vi "HovaCal Komm.vi"() -> (0 "error IO":errorcluster)   [LabVIEW 2020, in "Linearisierung v2.lvlib" / "Gasteiler.lvlib" / "HovaCal.lvlib"]
uses:
  HovaCal.lvlib
  Aktion_FGV_Kom.ctl
  Aktionen FGV Gasteiler Daten.ctl
  Daten abholen.ctl
  Aktion unterbrechen.ctl
  HovaCAL_Interface/Kommunikation/Aktion_FGV_HovaCAL_Interface_Kommunikation.ctl
  HovaCAL_Interface/Kommunikation/Aktion_FGV_HovaCAL_Interface_Kommandos.ctl
  Aktion FGV Stoerungen sammeln und auswerten.ctl
  Gasteiler.lvlib
  Linearisierung v2.lvlib
  Aktion FGV Rohmesswerte sammeln.ctl
  Aktion_FGV_Betriebsdaten.ctl
  Aktion Lin Daten aufarbeiten.ctl
  HovaCAL_Interface/Kommunikation/Kommunikation.lvlib
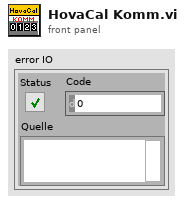
[diagram p1: front panel]
types:
  T1 = typedef "Linearisierung v2.lvlib/Gasteiler.lvlib/Aktion unterbrechen.ctl" = enum16{"Betrieb", "Unterbrechen", "Warten"}
  T2 = typedef "Linearisierung v2.lvlib/Daten abholen.ctl" = enum16{"Initialisieren", "Punkt aufschalten", "Warten", "Daten abholen", "Fertig", "Beenden", "Spülen", "Abbrechen"}
  T3 = typedef "Linearisierung v2.lvlib/Gasteiler.lvlib/Aktionen FGV Gasteiler Daten.ctl" = enum16{"lesen", "Gasteiler Daten", "Seriellen Param.", "MB-Endwert", "laden", "speichern", "Anforderung", "TCP", "Aufzeichnung Start"}
  T4 = typedef "Linearisierung v2.lvlib/Gasteiler.lvlib/HovaCal.lvlib/Aktion_FGV_Kom.ctl" = enum16{"Initialisieren", "Betriebsparameter", "Gase", "Vaporizer", "Dynamische Werte", "Beenden", "Com ändern", "Gase init"}
  T5 = typedef "Linearisierung v2.lvlib/Gasteiler.lvlib/HovaCAL_Interface.lvlib/Kommunikation.lvlib/Aktion_FGV_HovaCAL_Interface_Kommunikation.ctl" = enum16{"Initialisieren", "Set Konzentrationen", "Set Gase", "Set Limits", "Get Dynamische Werte", "Beenden", "Com ändern", "Get Gase init", "Pause", "Get Gasteiler Infos", "Get MFC Infos", "Set Pumpen Parameter", "Set Pumpe Konzenration", "Set Pumpe run", "Set Temperaturen", "Set Fluss", "Get Gase", "Get Limits", "Get Dynamische Werte 1", "Get Dynamische Werte 2"}
  T6 = typedef "Linearisierung v2.lvlib/Gasteiler.lvlib/HovaCAL_Interface.lvlib/Kommunikation.lvlib/Aktion_FGV_HovaCAL_Interface_Kommandos.ctl" = enum16{"lesen", "verarbeiten", "hinzufügen", "on top", "init", "sammeln", "freigeben", "connected"}
  T7 = typedef "Linearisierung v2.lvlib/Aktion Lin Daten aufarbeiten.ctl" = enum16{"lesen", "Protkolldaten", "speichern", "laden", "EPA auswerten", "Tabelle schreiben", "Lin auswerten", "Tab init", "Stufentabelle", "EPA aktiviert", "Nachbehandlung laden", "Tabelle löschen", "Istwerte löschen", "Zeile löschen", "Zeile einfügen", "LIN aktiviert", "LIN/EPA aktiv laden", "EGAK Tab", "LIN übernehmen", "Tab init ohne Stufen"}
  T8 = typedef "Linearisierung v2.lvlib/Gasteiler.lvlib/HovaCal.lvlib/Aktion_FGV_Betriebsdaten.ctl" = enum16{"Lesen", "Sollwerte schreiben", "Sollwerte lesen", "Gase schreiben", "Gase lesen", "Dynamische Werte", "GaseRef", "Gase aendern"}
  T9 = typedef "Linearisierung v2.lvlib/Aktion FGV Rohmesswerte sammeln.ctl" = enum16{"lesen", "schreiben", "löschen", "Sollwert HovaCal"}
  T10 = typedef "Linearisierung v2.lvlib/Aktion FGV Stoerungen sammeln und auswerten.ctl" = enum16{"init", "lesen", "error", "prüfen", "reset error", "abbrechen", "fortsetzen", "neustart", "Bedientasten reset"}
  T11 = typedef "Linearisierung v2.lvlib/Gasteiler.lvlib/Gasteiler Daten.ctl" = cluster{"Gasteiler":T12, "Gasteiler Stufen":T13, "Gasteiler Type":T14, "Konfig Gasteiler":T15, "Gasteiler Span Eingänge":u16}
  T12 = typedef "String - Eingabefeld.ctl" = string
  T13 = typedef "Linearisierung v2.lvlib/Gasteiler.lvlib/Gasteiler Stufen.ctl" = u16
  T14 = typedef "Linearisierung v2.lvlib/GasteilerType.ctl" = u16
  T15 = typedef "System Einstellungen V2.lvlib/Gasteiler Auswahl.ctl" = u16
  T16 = typedef "Linearisierung v2.lvlib/Lin-Polynom Daten.ctl" = cluster{"Messgerät":string, "Kalibrator (Gasteiler)":string, "Bearbeiter/in":string, "Komponente":string, "Zeitstempel":timestamp, "F_max gefordert (%)":sgl, "F_max in %":sgl, "F_max in ppm":sgl, "Vorschlag Ordnung":i32, "Polynom OK":bool, "Polynomkoeff.":dbl[], "Prüfgas Konzentration":dbl, "Pfad EPA":string, "Pfad_LIN":string, "Gasnummer:":u8, "Komponentenauswahl":T17, "Verdünnungsgas":T19, "Zeitdauer Stufe":T20, "Anzahl Stufen":T20, "F_max in % EPA":sgl, "F_max in ppm EPA":sgl, "F_max in % LIN":sgl, "F_max in ppm LIN":sgl, "Punkte umkehren":bool, "EPA Optionsfeld":T21, "Autolin Hovacal":T22, "Spanfactors":sgl[], "Kalibrierauswahl":T23, "Conditions:":T24, "Gasflaschen Nr.:":string, "Bottle Accuracy":dbl, "Konfig Gasflasche":T25, "Gasflasche":T26, "HovaCAL Flow AutoLin":T27, "MFC Output":T28, "Gas Ablaufdatum":timestamp, "Lin Modus":T29, "zusätzliche Zeitdauer Erster Punkt":sgl, "Offsets":sgl[]}
  T17 = typedef "Linearisierung v2.lvlib/KomponentenArray.ctl" = cluster{"Komponente:":T18, "Konzentration":dbl}[]
  T18 = typedef "Auswahlfeld.ctl" = u16
  T19 = typedef "Linearisierung v2.lvlib/Gasteiler.lvlib/Prüfgas in.ctl" = u16
  T20 = typedef "Zahlen-Eingabefeld.ctl" = sgl
  T21 = typedef "Linearisierung v2.lvlib/EPA Optionsfeld.ctl" = enum32{"Istwert", "Rohwert", "Linearisierter Wert"}
  T22 = typedef "Linearisierung v2.lvlib/Gasteiler.lvlib/HovaCal.lvlib/AutoLin Hovacal.ctl" = enum32{"Keine Auswahl", "Optionsauswahl 1", "Optionsauswahl 2"}
  T23 = typedef "Linearisierung v2.lvlib/Kalibrieroption.ctl" = u16
  T24 = typedef "Linearisierung v2.lvlib/Linearity verification 1065-307.lvlib/Condition.ctl" = u16
  T25 = typedef "System Einstellungen V2.lvlib/Konfig Gasflasche.ctl" = bool
  T26 = typedef "System Einstellungen V2.lvlib/Gasflasche Auswahl.ctl" = u16
  T27 = typedef "Linearisierung v2.lvlib/Gasteiler.lvlib/HovaCAL_Interface.lvlib/Controls.lvlib/Flow Einstellung.ctl" = cluster{"HovaCAL Flow Input Cluster":dbl}
  T28 = typedef "Linearisierung v2.lvlib/Gasteiler.lvlib/HovaCAL_Interface.lvlib/Controls.lvlib/Pump state.ctl" = cluster{"Run":bool}
  T29 = typedef "CalGas Aufschaltung.lvlib/Lin Modus.ctl" = u16
  T30 = typedef "Linearisierung v2.lvlib/Gasteiler.lvlib/HovaCal.lvlib/Dynamsiche_Werte.ctl" = cluster{"Durchfluss":dbl, "Drehzahl":dbl, "Wasserkonz.":dbl, "Ist - Temp":dbl, "Ist Konz 1":dbl, "Ist Konz 2":dbl}
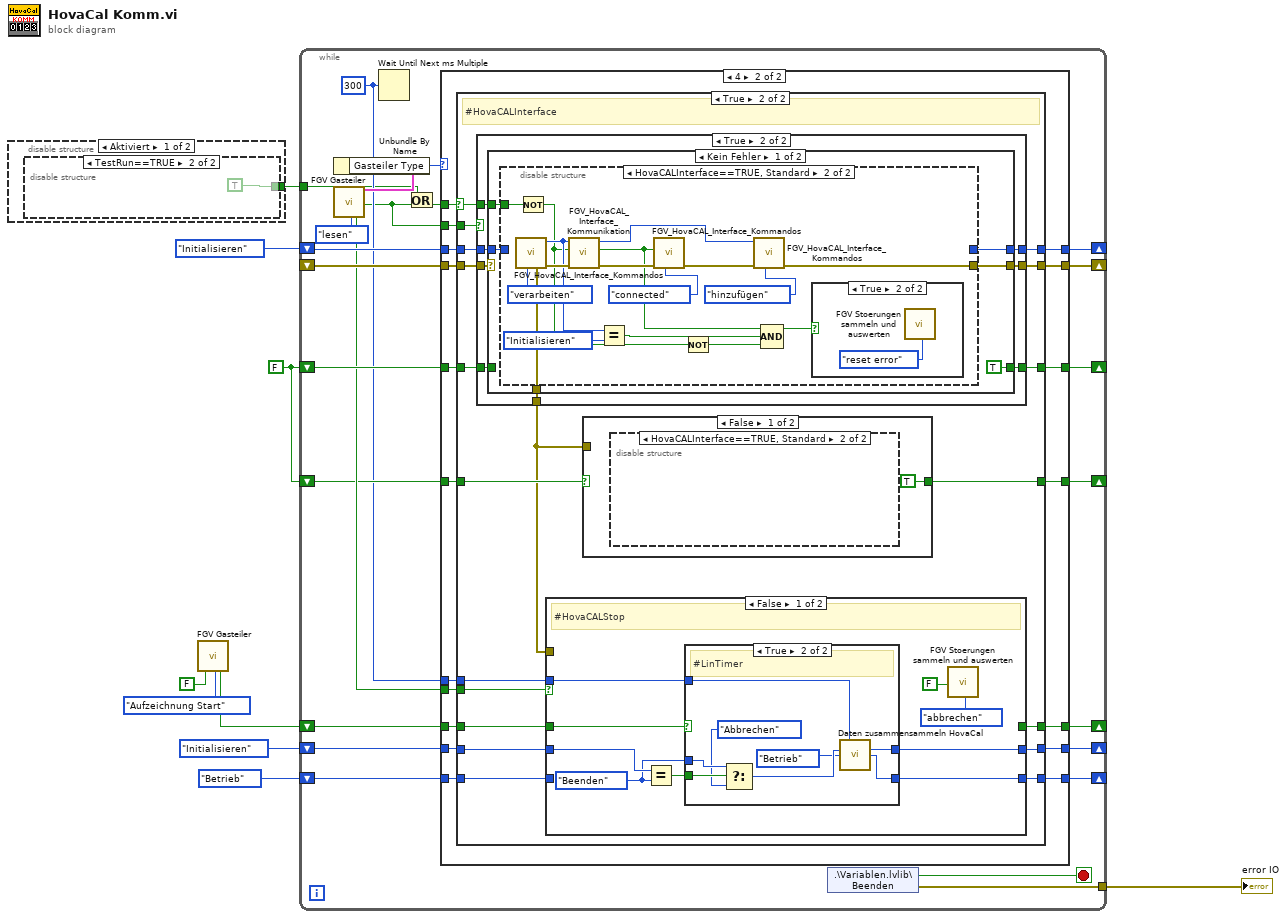
[diagram p0: block diagram]
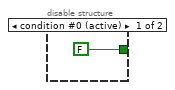
[diagram p2: hidden frame]
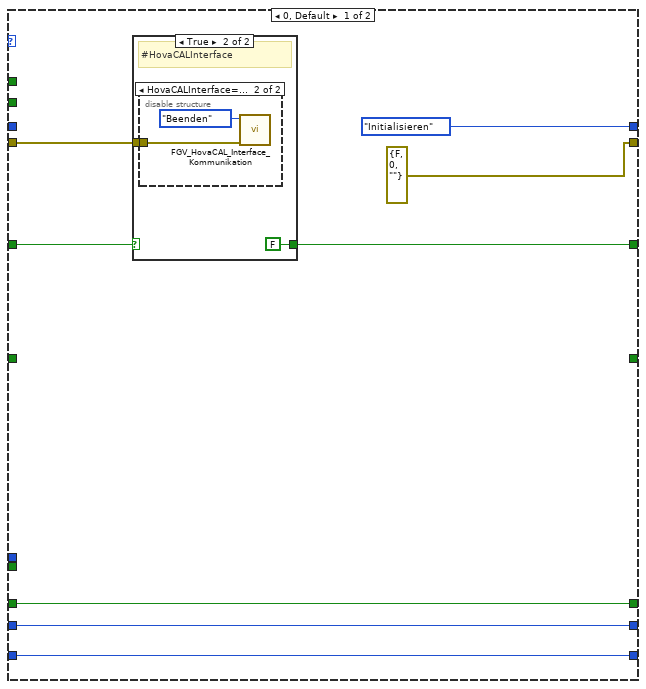
[diagram p4: hidden frame]
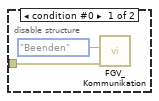
[diagram p6: hidden frame]
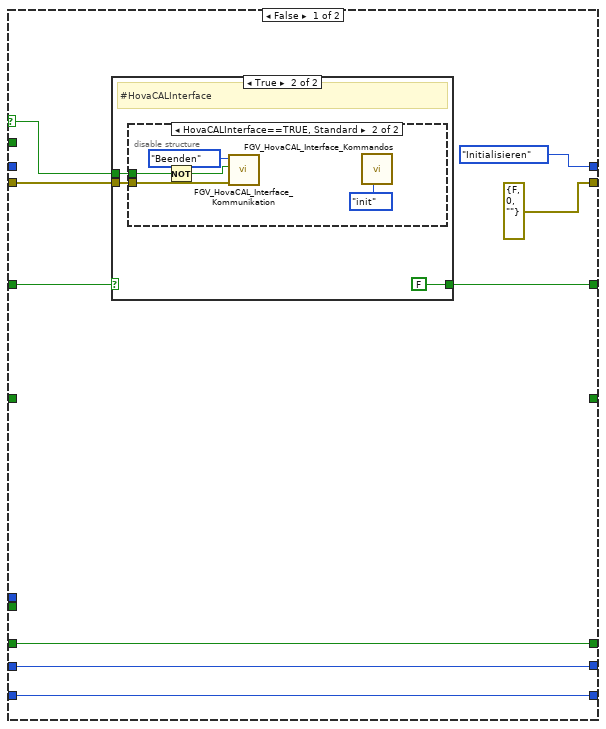
[diagram p7: hidden frame]
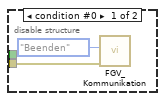
[diagram p9: hidden frame]
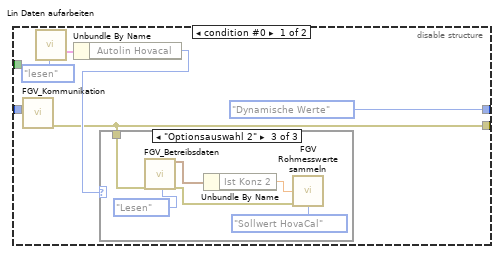
[diagram p11: hidden frame]
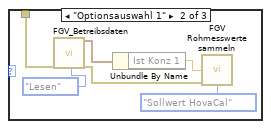
[diagram p13: hidden frame]
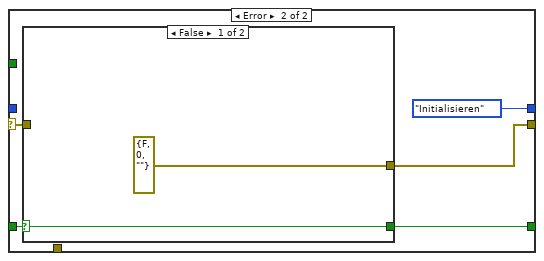
[diagram p15: hidden frame]
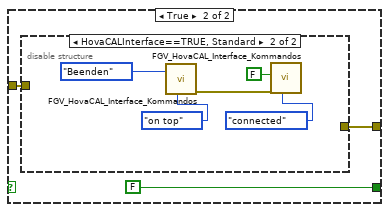
[diagram p16: hidden frame]
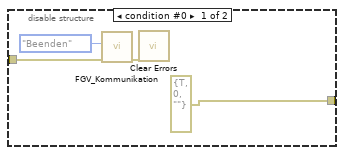
[diagram p17: hidden frame]
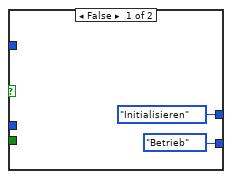
[diagram p18: hidden frame]
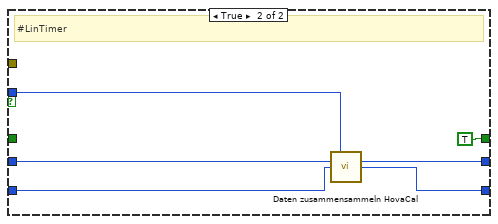
[diagram p19: hidden frame]
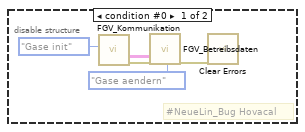
[diagram p20: hidden frame]
diagram:
  w4 = FALSE
  n1 = disable-structure shown="Aktiviert" {
    disable-tunnel: [w10 _] -> w2
    frame Enabled {
      n2 = disable-structure shown="TestRun==TRUE" {
        disable-tunnel: [FALSE TRUE] -> w10
        frame condition #0 (active) {
        }
        frame condition #1 {
        }
      }
    }
    frame Disabled {
    }
  }
  n3 = call "FGV Gasteiler.vi"("Aufzeichnung Start"=FALSE, "Aktionen"=Aktionen_FGV_Gasteiler_Daten."Aufzeichnung Start") -> ("Aufzeichnung Start"=w5:bool)  [unwired: 10 in, 7 out]
  n4 = while {
    shift-right: [w35] -> _
    shift-left: Aktion_FGV_Kom."Initialisieren" ("Aktion") -> [w36]
    shift-right: [w33] -> _
    shift-left: _ -> [w32]
    tunnel: [w30] -> w8
    shift-right: [w27] -> _
    shift-left: w4 -> [w28]
    shift-right: [w26] -> _
    shift-left: w5 -> [w25]
    shift-right: [w23] -> _
    shift-left: Daten_abholen."Initialisieren" ("Aktionen Daten abholen") -> [w24]
    shift-right: [w20] -> _
    shift-left: w4 -> [w21]
    tunnel: w2 -> [w16]
    shift-right: [w13] -> _
    shift-left: Aktion_unterbrechen."Betrieb" ("Aktion Unterbrechen") -> [w14]
    stop <- w31 stop-if-true
    w18 = u32 300 ("Vielfache von ms")
    n5 = call "FGV Gasteiler.vi"("Aktionen"=Aktionen_FGV_Gasteiler_Daten."lesen") -> ("Aufzeichnung Start"=w22:bool, "Gasteiler Daten"=w29:T11, "Anforderung"=w15:bool)  [unwired: 11 in, 5 out]
    n6 = Unbundle By Name(w29) -> ("Gasteiler Type"=w19:T14)
    n7 = Wait Until Next ms Multiple(millisecond multiple=w18) -> ()  [unwired: 1 out]
    n8 = Or(x=w16, y=w15) -> (x .or. y?=w17:bool)
    n9 = case shown="4" w19 {
      tunnel: w36 -> [_ w69]
      tunnel: [Aktion_FGV_Kom."Initialisieren" ("Aktion") w68] -> w35
      tunnel: w17 -> [_ w67]
      tunnel: [errorcluster {"status"=FALSE, "code"=0, "source"=""} ("error out") w66] -> w33
      tunnel: w32 -> [w40 w65]
      tunnel: w28 -> [w42 w64]
      tunnel: [w41 w63] -> w27
      tunnel: [w39 w56] -> w26
      tunnel: w25 -> [w39 w58]
      tunnel: w24 -> [w38 w59]
      tunnel: [w38 w57] -> w23
      tunnel: w22 -> [_ w60]
      tunnel: w21 -> [_ w62]
      tunnel: [_ w61] -> w20
      tunnel: w18 -> [_ w55]
      tunnel: w15 -> [_ w54]
      tunnel: w14 -> [w37 w53]
      tunnel: [w37 w52] -> w13
      frame 0, Default {
        n10 = case shown="True" w42 {
          selector: w42 -> [w45 _]
          tunnel: w40 -> [_ w47]
          tunnel: [w45 FALSE] -> w41
          frame False {
          }
          frame True {
            # "#HovaCALInterface"
            n11 = disable-structure shown="HovaCALInterface==TRUE, Standard" {
              disable-tunnel: w47 -> [w49 w50]
              frame condition #0 {
                n12 = call "FGV_Kommunikation.vi"("error in"=w49, "Aktion"=Aktion_FGV_Kom."Beenden") -> ()  [unwired: 5 in, 5 out]
              }
              frame condition #1 (active) {
                n13 = call "FGV_HovaCAL_Interface_Kommunikation.vi"("error in"=w50, "Aktion"=Aktion_FGV_HovaCAL_Interface_Kommunikation."Beenden") -> ()  [unwired: 7 in, 3 out]
              }
            }
          }
        }
      }
      frame 4 {
        n14 = case shown="True" w67 {
          selector: w67 -> [w71 w95]
          tunnel: w69 -> [_ w108]
          tunnel: [Aktion_FGV_Kom."Initialisieren" ("Aktion") w107] -> w68
          tunnel: [errorcluster {"status"=FALSE, "code"=0, "source"=""} ("error out") w92] -> w66
          tunnel: w65 -> [w74 w106]
          tunnel: w64 -> [w76 w105]
          tunnel: [w75 w104] -> w63
          tunnel: w62 -> [_ w103]
          tunnel: [_ w102] -> w61
          tunnel: w60 -> [_ w101]
          tunnel: w59 -> [w72 w100]
          tunnel: w58 -> [w73 w99]
          tunnel: [w72 w98] -> w57
          tunnel: [w73 w97] -> w56
          tunnel: w55 -> [_ w94]
          tunnel: w54 -> [_ w93]
          tunnel: w53 -> [w70 w91]
          tunnel: [w70 w90] -> w52
          frame False {
            n15 = case shown="True" w76 {
              selector: w76 -> [w79 _]
              tunnel: w74 -> [_ w81]
              tunnel: [w79 FALSE] -> w75
              tunnel: w71 -> [_ w80]
              frame False {
              }
              frame True {
                # "#HovaCALInterface"
                n16 = disable-structure shown="HovaCALInterface==TRUE, Standard" {
                  disable-tunnel: w81 -> [w84 w88]
                  disable-tunnel: w80 -> [_ w86]
                  frame condition #0 {
                    n17 = call "FGV_Kommunikation.vi"("error in"=w84, "Aktion"=Aktion_FGV_Kom."Beenden") -> ()  [unwired: 5 in, 5 out]
                  }
                  frame condition #1 (active) {
                    n18 = Not(x=w86) -> (.not. x?=w85:bool)
                    n19 = call "FGV_HovaCAL_Interface_Kommunikation.vi"("error in"=w88, "Stop"=w85, "Aktion"=Aktion_FGV_HovaCAL_Interface_Kommunikation."Beenden") -> ()  [unwired: 6 in, 3 out]
                    n20 = call "FGV_HovaCAL_Interface_Kommandos.vi"("Aktion"=Aktion_FGV_HovaCAL_Interface_Kommandos."init") -> ()  [unwired: 4 in, 6 out]
                  }
                }
              }
            }
          }
          frame True {
            # "#HovaCALInterface"
            n21 = case shown="True" w93 {
              tunnel: w108 -> [w111 w119]
              tunnel: [w111 w118] -> w107
              tunnel: w106 -> [w109 w116]
              tunnel: w105 -> [w110 w115]
              tunnel: [w110 w114] -> w104
              tunnel: [w109 w113] -> w96
              tunnel: w95 -> [_ w112]
              tunnel: [w109 w117] -> w92
              frame False {
              }
              frame True {
                n22 = case shown="Kein Fehler" w116 {
                  selector: w116 -> [_ w164]
                  tunnel: w119 -> [w124 _]
                  tunnel: [w123 Aktion_FGV_Kom."Initialisieren" ("Aktion")] -> w118
                  tunnel: [w122 w160] -> w117
                  tunnel: w115 -> [_ w163]
                  tunnel: [TRUE w162] -> w114
                  tunnel: [w122 _] -> w113
                  tunnel: w112 -> [w120 _]
                  frame No Error {
                    n23 = disable-structure shown="HovaCALInterface==TRUE, Standard" {
                      disable-tunnel: w124 -> [w130 _]
                      disable-tunnel: [Aktion_FGV_Kom."Dynamische Werte" ("Aktion") _] -> w123
                      disable-tunnel: [w125 w155] -> w122
                      disable-tunnel: w120 -> [_ w154]
                      frame condition #0 {
                        n24 = call "FGV_Kommunikation.vi"("Aktion"=w130) -> ("error out"=w125:errorcluster)  [unwired: 6 in, 4 out]
                        n25 = call "Lin Daten aufarbeiten.vi"("Aktionen"=Aktion_Lin_Daten_aufarbeiten."lesen") -> ("Lin-Polynom"=w127:T16)  [unwired: 16 in, 10 out]
                        n26 = Unbundle By Name(w127) -> ("Autolin Hovacal"=w126:T22)
                        n27 = case shown="\"Optionsauswahl 2\"" w126 {
                          tunnel: w125 -> [_ w135 w141]
                          frame "Keine Auswahl", Default {
                          }
                          frame "Optionsauswahl 1" {
                            n28 = call "FGV_Betreibsdaten.vi"("error in (no error)"=w135, "Enum"=Aktion_FGV_Betriebsdaten."Lesen" ("Aktion")) -> ("Dynamische Werte 2"=w133:T30, "error out"=w134:errorcluster)  [unwired: 10 in, 6 out]
                            n29 = Unbundle By Name(w133) -> ("Ist Konz 1"=w132:dbl)
                            n30 = call "FGV Rohmesswerte sammeln.vi"("Sollwert"=w132, "error in (no error)"=w134, "Aktion"=Aktion_FGV_Rohmesswerte_sammeln."Sollwert HovaCal") -> ()  [unwired: 9 in, 4 out]
                          }
                          frame "Optionsauswahl 2" {
                            n31 = call "FGV_Betreibsdaten.vi"("error in (no error)"=w141, "Enum"=Aktion_FGV_Betriebsdaten."Lesen" ("Aktion")) -> ("Dynamische Werte 2"=w139:T30, "error out"=w140:errorcluster)  [unwired: 10 in, 6 out]
                            n32 = Unbundle By Name(w139) -> ("Ist Konz 2"=w138:dbl)
                            n33 = call "FGV Rohmesswerte sammeln.vi"("Sollwert"=w138, "error in (no error)"=w140, "Aktion"=Aktion_FGV_Rohmesswerte_sammeln."Sollwert HovaCal") -> ()  [unwired: 9 in, 4 out]
                          }
                        }
                      }
                      frame condition #1 (active) {
                        n34 = call "FGV_HovaCAL_Interface_Kommandos.vi"("Aktion"=Aktion_FGV_HovaCAL_Interface_Kommandos."verarbeiten") -> ("error out"=w156:errorcluster, "Kommando out"=w147:T5)  [unwired: 4 in, 4 out]
                        n35 = Not(x=w154) -> (.not. x?=w144:bool)
                        n36 = call "FGV_HovaCAL_Interface_Kommunikation.vi"("error in"=w156, "Stop"=w144, "Aktion"=w147) -> ("error out"=w152:errorcluster, "connected?"=w149:bool, "Aktion out"=w150:T5)  [unwired: 6 in]
                        n37 = Equal?(x=w147, y=Aktion_FGV_HovaCAL_Interface_Kommunikation."Initialisieren") -> (x = y?=w145:bool)
                        n38 = call "FGV_HovaCAL_Interface_Kommandos.vi"("Aktion"=Aktion_FGV_HovaCAL_Interface_Kommandos."connected", "error in"=w152, "connected in ?"=w149) -> ("error out"=w151:errorcluster)  [unwired: 2 in, 5 out]
                        n39 = Not(x=w144) -> (.not. x?=w143:bool)
                        n40 = call "FGV_HovaCAL_Interface_Kommandos.vi"("Aktion"=Aktion_FGV_HovaCAL_Interface_Kommandos."hinzufügen", "error in"=w151, "Kommando in"=w150) -> ("error out"=w155:errorcluster)  [unwired: 2 in, 5 out]
                        n41 = Compound Arithmetic op=AND ("Mehrfacharithmetik")(w149, w145, w143) -> (w148:bool)
                        n42 = case shown="True" w148 {
                          frame False {
                          }
                          frame True {
                            n43 = call "FGV Stoerungen sammeln und auswerten.vi"("Aktion"=Aktion_FGV_Stoerungen_sammeln_und_auswerten."reset error") -> ()  [unwired: 12 in, 7 out]
                          }
                        }
                      }
                    }
                  }
                  frame Error {
                    n44 = case shown="False" w163 {
                      selector: w163 -> [w165 _]
                      tunnel: w164 -> [_ w169]
                      tunnel: [w165 FALSE] -> w162
                      tunnel: [errorcluster {"status"=FALSE, "code"=0, "source"=""} ("error out") w167] -> w160
                      frame False {
                      }
                      frame True {
                        n45 = disable-structure shown="HovaCALInterface==TRUE, Standard" {
                          disable-tunnel: w169 -> [w173 _]
                          disable-tunnel: [errorcluster {"status"=TRUE, "code"=0, "source"=""} ("error out") _] -> w167
                          frame condition #0 {
                            n46 = call "FGV_Kommunikation.vi"("error in"=w173, "Aktion"=Aktion_FGV_Kom."Beenden") -> ("error out"=w171:errorcluster)  [unwired: 5 in, 4 out]
                            n47 = call <vilib>:"Clear Errors.vi"("error in (no error)"=w171) -> ()  [unwired: 5 in, 2 out]
                          }
                          frame condition #1 (active) {
                            n48 = call "FGV_HovaCAL_Interface_Kommandos.vi"("Aktion"=Aktion_FGV_HovaCAL_Interface_Kommandos."on top", "Kommando in"=Aktion_FGV_HovaCAL_Interface_Kommunikation."Beenden") -> ("error out"=w175:errorcluster)  [unwired: 3 in, 5 out]
                            n49 = call "FGV_HovaCAL_Interface_Kommandos.vi"("Aktion"=Aktion_FGV_HovaCAL_Interface_Kommandos."connected", "error in"=w175, "connected in ?"=FALSE) -> ()  [unwired: 2 in, 6 out]
                          }
                        }
                      }
                    }
                  }
                }
              }
            }
            n50 = case shown="False" w101 {
              tunnel: w100 -> [w185 w203]
              tunnel: [w187 w202] -> w98
              tunnel: w99 -> [w186 _]
              tunnel: [_ TRUE ("Aufzeichnung Start")] -> w97
              tunnel: w96 -> [_ _]
              tunnel: w94 -> [w182 w200]
              tunnel: w91 -> [_ w199]
              tunnel: [w179 w198] -> w90
              frame False {
                w183 = Daten_abholen."Beenden" ("y")
                # "#HovaCALStop"
                n51 = Equal?(x=w185, y=w183) -> (x = y?=w184:bool)
                n52 = case shown="True" w186 {
                  tunnel: [Daten_abholen."Initialisieren" ("Aktionen Daten abholen") w197] -> w187
                  tunnel: w184 -> [_ w196]
                  tunnel: w183 -> [_ w195]
                  tunnel: w182 -> [_ w192]
                  tunnel: [Aktion_unterbrechen."Betrieb" ("Aktion Unterbrechen") w190] -> w179
                  frame False {
                  }
                  frame True {
                    # "#LinTimer"
                    n53 = Select(t=w195, s=w196, f=Daten_abholen."Abbrechen" ("Aktionen Daten abholen")) -> (s? t:f=w194:T2)
                    n54 = call "Daten zusammensammeln HovaCal.vi"("KommLoopTimer"=w192, "Aktionen Daten abholen"=w194, "Aktion Unterbrechen"=Aktion_unterbrechen."Betrieb") -> ("Aktionen Daten abholen"=w197:T2, "Aktion Unterbrechen out"=w190:T1)  [unwired: 8 in, 3 out]
                  }
                }
                n55 = call "FGV Stoerungen sammeln und auswerten.vi"("Abbrechen"=FALSE, "Aktion"=Aktion_FGV_Stoerungen_sammeln_und_auswerten."abbrechen") -> ()  [unwired: 11 in, 7 out]
              }
              frame True {
                # "#LinTimer"
                n56 = call "Daten zusammensammeln HovaCal.vi"("KommLoopTimer"=w200, "Aktionen Daten abholen"=w203, "Aktion Unterbrechen"=w199) -> ("Aktionen Daten abholen"=w202:T2, "Aktion Unterbrechen out"=w198:T1)  [unwired: 8 in, 3 out]
              }
            }
            n57 = case shown="False" w103 {
              selector: w103 -> [_ w210]
              tunnel: [TRUE w210] -> w102
              tunnel: w96 -> [_ _]
              frame False {
                n58 = disable-structure shown="HovaCALInterface==TRUE, Standard" {
                  frame condition #0 {
                    # "#NeueLin_Bug Hovacal"
                    n59 = call "FGV_Kommunikation.vi"("Aktion"=Aktion_FGV_Kom."Gase init") -> ("error out"=w208:errorcluster, "Gase"=w206:cluster{string, i32}[][])  [unwired: 6 in, 3 out]
                    n60 = call "FGV_Betreibsdaten.vi"("Strings und Werte"=w206, "error in (no error)"=w208, "Enum"=Aktion_FGV_Betriebsdaten."Gase aendern") -> ("error out"=w207:errorcluster)  [unwired: 9 in, 7 out]
                    n61 = call <vilib>:"Clear Errors.vi"("error in (no error)"=w207) -> ()  [unwired: 5 in, 2 out]
                  }
                  frame condition #1 (active) {
                  }
                }
              }
              frame True {
              }
            }
          }
        }
      }
    }
    n62 = shared-variable ".\\Variablen.lvlib\\Beenden"() -> (w31:bool, error out=w30:errorcluster)  [unwired: 1 out]
  }
  "error IO" <- w8
